vi "保存.vi"(8 "error in (no error)":errorcluster caption="错误输入（无错误）", 11 "数据文件.lvclass":refnum<class "数据文件.lvclass">) -> (0 "error out":errorcluster caption="错误输出", 3 "数据文件.lvclass":refnum<class "数据文件.lvclass">)   [LabVIEW 2021, in "数据文件.lvclass"]
doc: "本VI是为《我和LabVIEW》一书编写的示例。\n关于本书的介绍请参考网页：\nhttp://ruanqizhen.spaces.live.com/blog/cns!5852D4F797C53FB6!4310.entry"
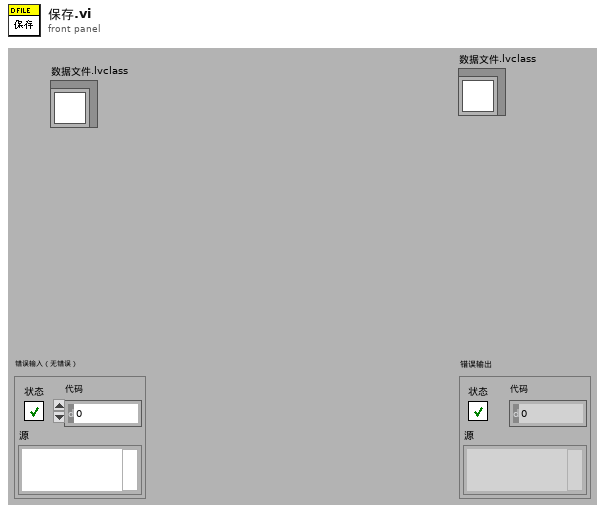
[diagram p1: front panel]
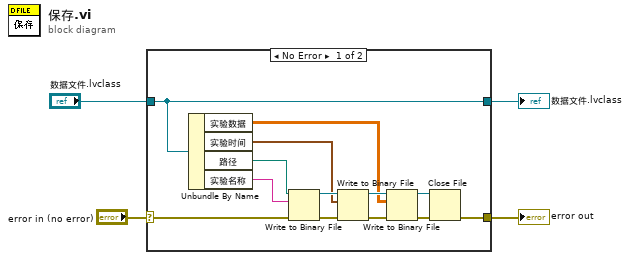
[diagram p0: block diagram]
diagram:
  n1 = case shown="No Error" "error in (no error)" {
    selector: "error in (no error)" -> [w17 w19]
    tunnel: [w16 w19] -> w3
    tunnel: [w8 w18] -> w1
    tunnel: "数据文件.lvclass" -> [w8 w18]
    frame No Error {
      n2 = Unbundle By Name(w8) -> ("实验数据"=w5:dbl[][], "实验时间"=w6:timestamp, "路径"=w9:path, "实验名称"=w7:string)
      n3 = Write to Binary File(file (use dialog)=w9, data=w7, error in=w17) -> (refnum out=w14:refnum<file>, error out=w13:errorcluster)  [unwired: 1 in, 3 out]
      n4 = Write to Binary File(file (use dialog)=w14, data=w6, error in=w13) -> (refnum out=w15:refnum<file>, error out=w12:errorcluster)  [unwired: 1 in, 3 out]
      n5 = Write to Binary File(file (use dialog)=w15, data=w5, error in=w12) -> (refnum out=w11:refnum<file>, error out=w10:errorcluster)  [unwired: 1 in, 3 out]
      n6 = Close File(refnum=w11, error in=w10) -> (error out=w16:errorcluster)  [unwired: 1 out]
    }
    frame Error {
    }
  }
  "error out" <- w3
  "数据文件.lvclass" <- w1
